vi "repPrepareGoalKickAllyPlayVSS.vi"(8 "error in (no error)":errorcluster, 9 "Game in 2":refnum<class "Game.lvclass">, 10 "RobotPlacement":T1(array[cluster]), 11 "PrepareGoalKickAllyPlayVSS in":refnum<class "PrepareGoalKickAllyPlayVSS.lvclass">) -> (0 "error out":errorcluster, 2 "RobotPlacement 2":T1(array[cluster]), 3 "PrepareGoalKickAllyPlayVSS out":refnum<class "PrepareGoalKickAllyPlayVSS.lvclass">)   [LabVIEW 2023, in "PrepareGoalKickAllyPlayVSS.lvclass"]
uses:
  PrepareGoalKickAllyPlayVSS.lvclass
  Game_class/Game.lvclass
  Game_class/Game.lvclass/Game.ctl
  Game_class/Read FieldRef.vi
  Field_class/Field.lvclass
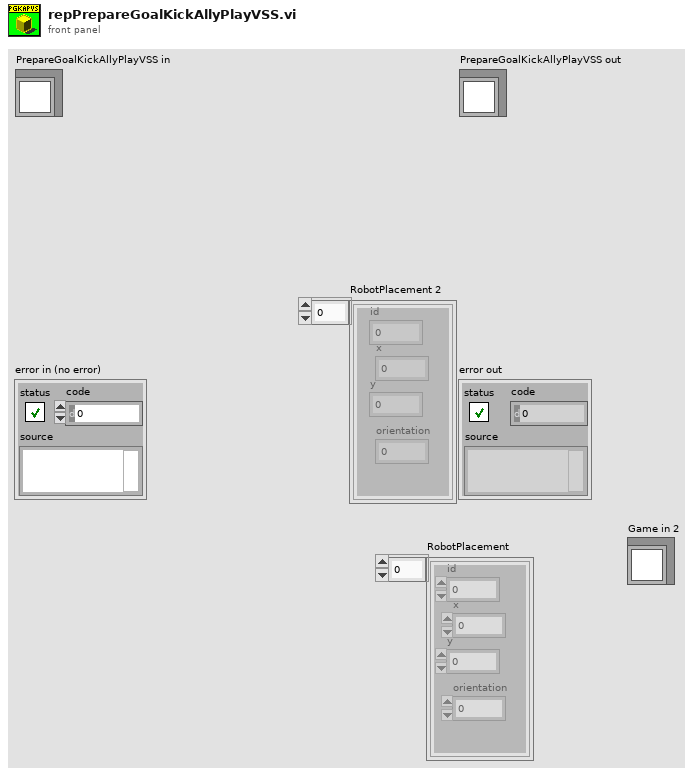
[diagram p1: front panel]
types:
  T1 = cluster{"id":i32, "x":dbl, "y":dbl, "orientation":dbl}[]
  T2 = cluster{"id":i32, "x":dbl, "y":dbl, "orientation":dbl}
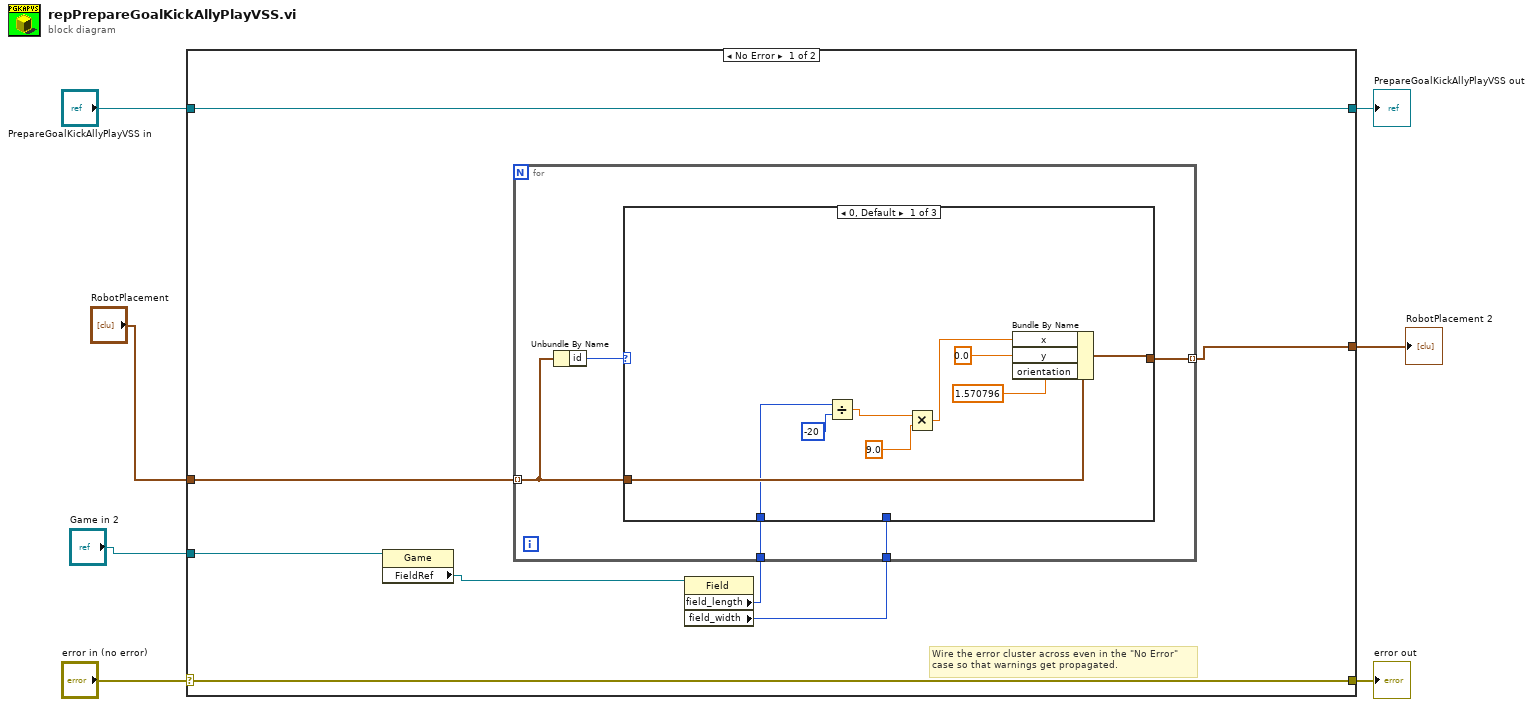
[diagram p0: block diagram]
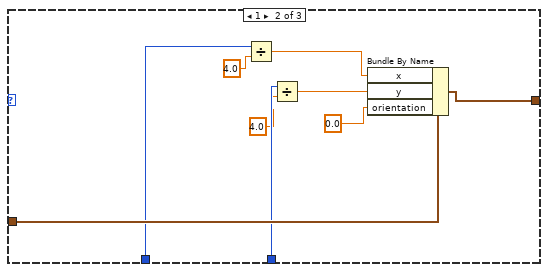
[diagram p2: hidden frame]
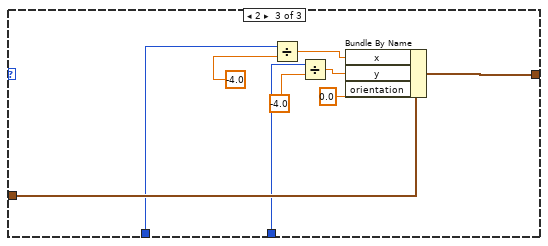
[diagram p3: hidden frame]
diagram:
  n1 = case shown="No Error" "error in (no error)" {
    selector: "error in (no error)" -> [w14 w49]
    tunnel: [w14 w49] -> w6
    tunnel: [w15 w48] -> w4
    tunnel: "PrepareGoalKickAllyPlayVSS in" -> [w15 w48]
    tunnel: [w13 _] -> w3
    tunnel: "RobotPlacement" -> [w12 _]
    tunnel: "Game in 2" -> [w11 _]
    frame No Error {
      # "Wire the error cluster across even in the \"No Error\"\ncase so that warnings get propagated."
      n2 = property class="Game"(reference=w11) -> ("FieldRef"=w10:refnum<class "Field.lvclass">)  [unwired: 1 in, 2 out]
      n3 = property class="Field"(reference=w10) -> ("field_length"=w9:i32, "field_width"=w8:i32)  [unwired: 1 in, 2 out]
      n4 = for {
        tunnel: [w20] -> w13 mode=indexing
        tunnel: w12 -> [w18] mode=indexing
        tunnel: w9 -> [w17]
        tunnel: w8 -> [w16]
        n5 = Unbundle By Name(w18) -> ("id"=w19:i32)
        n6 = case shown="0, Default" w19 {
          tunnel: [w29 w37 w47] -> w20
          tunnel: w18 -> [w25 w36 w45]
          tunnel: w17 -> [w24 w31 w39]
          tunnel: w16 -> [_ w35 w42]
          frame 0, Default {
            n7 = Divide(x=w24, y=-20) -> (x/y=w23:dbl)
            n8 = Multiply(x=w23, y=9.0) -> (x*y=w21:dbl)
            n9 = Bundle By Name(cluster=w25, "x"=w21, "y"=0.0, "orientation"=1.570796) -> (w29:T2)
          }
          frame 1 {
            n10 = Divide(x=w31, y=4.0 ("x")) -> (x/y=w30:dbl)
            n11 = Divide(x=w35, y=4.0 ("x")) -> (x/y=w32:dbl)
            n12 = Bundle By Name(cluster=w36, "x"=w30, "y"=w32, "orientation"=0.0 ("x")) -> (w37:T2)
          }
          frame 2 {
            n13 = Divide(x=w39, y=-4.0 ("x")) -> (x/y=w40:dbl)
            n14 = Divide(x=w42, y=-4.0 ("x")) -> (x/y=w41:dbl)
            n15 = Bundle By Name(cluster=w45, "x"=w40, "y"=w41, "orientation"=0.0) -> (w47:T2)
          }
        }
      }
    }
    frame Error {
    }
  }
  "error out" <- w6
  "PrepareGoalKickAllyPlayVSS out" <- w4
  "RobotPlacement 2" <- w3
